vi "Tools Panel.vi"() -> ()   [LabVIEW 2019, in "Panther Dashboard.lvlib"]
uses:
  Panther Dashboard.lvlib
  <vilib>/PantherLAB/Panther Dashboard/Controls/Antidoc.ctl
  DQMH Tools Menu--enum.ctl
panel:
  in  "Add Event":bool caption="Add"
  in  "Remove Event":bool caption="Remove"
  in  "Convert Event":bool caption="Convert"
  in  "Rename Event":bool caption="Rename"
  in  "Open Documentation":bool caption="Open"
  in  "Generate Antidoc":T1 caption="Antidoc"
  in  "Add Module":bool caption="Add"
  in  "Rename Module":bool caption="Rename"
  in  "Validate Module":bool caption="Validate"
  in  "Create Module Template":bool caption="Template"
  in  "Add Unit Test":bool caption="Unit Test"
  in  "Create RT Tester":bool caption="RT Tester"
  in  "About":bool
  in  "Theme":bool
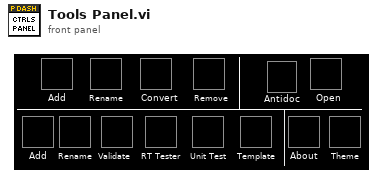
[diagram p1: front panel]
types:
  T1 = typedef "Antidoc.ctl" = bool
  T2 = typedef "Panther Dashboard.lvlib/Broadcast Events--cluster.ctl" = cluster{"Module Did Init":refnum<user-event>, "Status Updated":refnum<user-event>, "Error Reported":refnum<user-event>, "Module Did Stop":refnum<user-event>, "Update Module Execution Status":refnum<user-event>, "References Updated":refnum<user-event>, "Projects Updated":refnum<user-event>, "Targets Updated":refnum<user-event>, "Progress updated":refnum<user-event>, "Scale Updated":refnum<user-event>, "Connector Pane Updated":refnum<user-event>, "Documentation Updated":refnum<user-event>, "Module Type Updated":refnum<user-event>, "Theme Updated":refnum<user-event>, "Panel Position Updated":refnum<user-event>}
  T3 = typedef "Panther Dashboard.lvlib/DQMH Tools Menu--enum.ctl" = enum16{"Create New DQMH Event", "Remove DQMH Event", "Convert DQMH Event", "Rename DQMH Event", "Add New DQMH Module", "Create RT Tester", "Rename DQMH Module", "Validate DQMH Module", "Create DQMH Module Template", "New DQMH  Unit Test"}
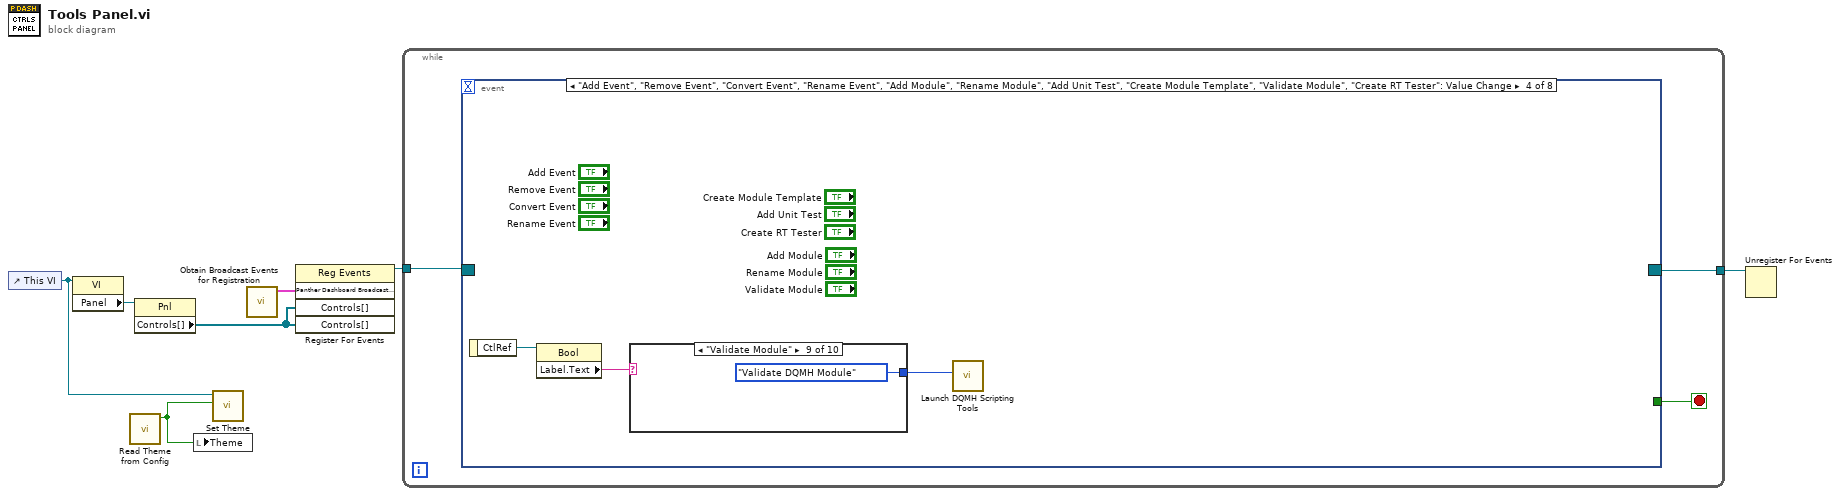
[diagram p0: block diagram]
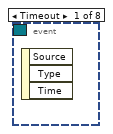
[diagram p2: hidden frame]
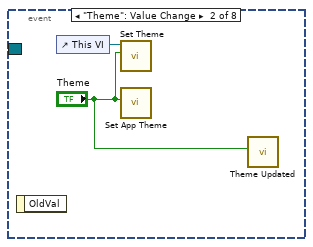
[diagram p3: hidden frame]
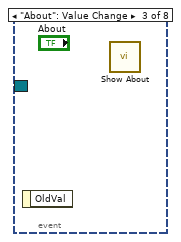
[diagram p4: hidden frame]
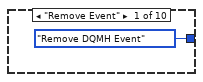
[diagram p5: hidden frame]
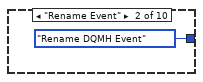
[diagram p6: hidden frame]
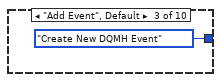
[diagram p7: hidden frame]
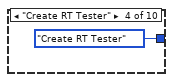
[diagram p8: hidden frame]
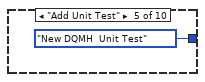
[diagram p9: hidden frame]
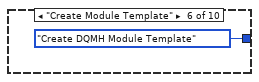
[diagram p10: hidden frame]
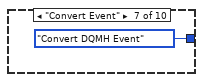
[diagram p11: hidden frame]
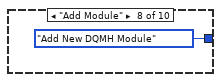
[diagram p12: hidden frame]
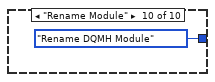
[diagram p13: hidden frame]
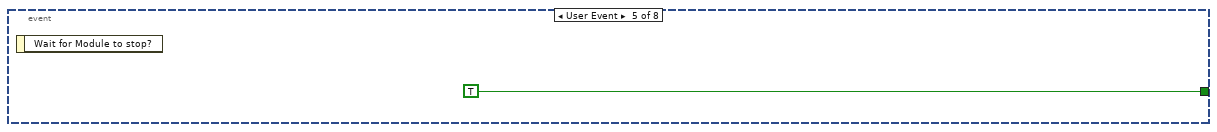
[diagram p14: hidden frame]
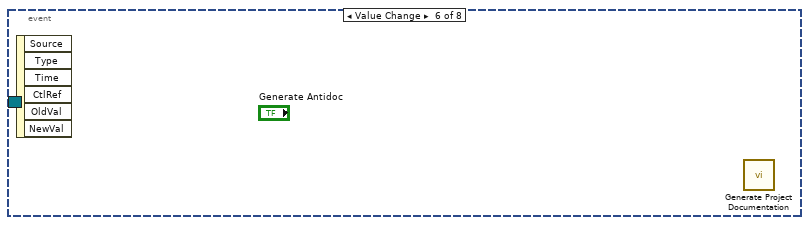
[diagram p15: hidden frame]
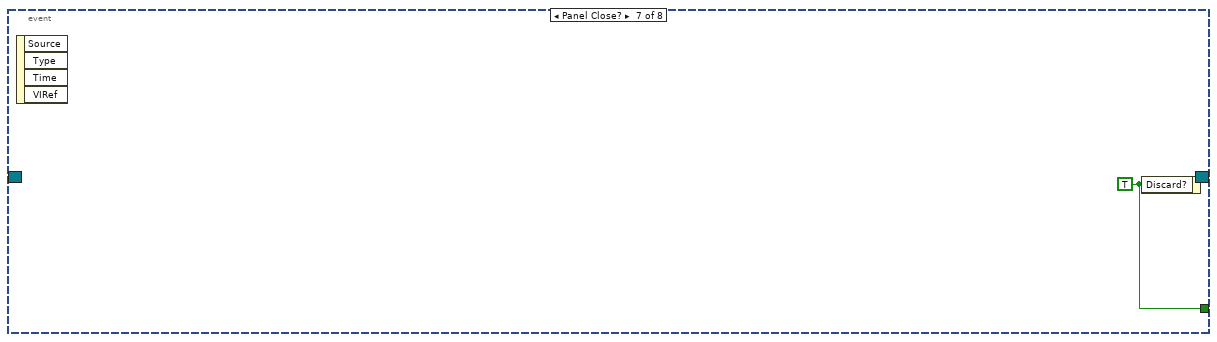
[diagram p16: hidden frame]
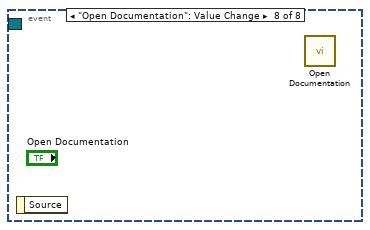
[diagram p17: hidden frame]
diagram:
  n1 = control-ref of="This VI"() -> (w4:refnum<vi>)
  n2 = property class="VI"(reference=w4) -> ("Panel"=w3:refnum<vi>)  [unwired: 1 in, 2 out]
  n3 = call "Read Theme from Config.vi"() -> ("Theme"=w1:bool)  [unwired: 10 in, 1 out]
  n4 = property class="Pnl"(reference=w3) -> ("Controls[]"=w2:refnum<vi>[])  [unwired: 1 in, 2 out]
  n5 = local write "Theme"(w1) -> ()
  n6 = call "Set Theme.vi"("Dark?"=w1, "VI in"=w4) -> ()  [unwired: 10 in]
  n7 = call "Obtain Broadcast Events for Registration.vi"() -> ("Panther Dashboard Broadcast Events"=w6:T2)  [unwired: 9 in, 2 out]
  n8 = register-events(w6, w2, w2) -> (reference out=w7:refnum<event-registration>)  [unwired: 2 in, 1 out]
  n9 = while {
    tunnel: w7 -> [w10]
    tunnel: [w8] -> w5
    stop <- w9 stop-if-true
    n10 = event shown="[3] \"Add Event\", \"Remove Event\", \"Convert Event\", \"Rename Event\", \"Add Module\", \"Rename Module\", \"Add Unit Test\", \"Create Module Template\", \"Validate Module\", \"Create RT Tester\": Value Change" {
      selector: w10 -> [_ _ _ _ _ _ _ _]
      dyn-events: [_ _ _ _ _ _ _ _] -> w8
      timeout: _ -> [_ _ _ _ _ _ _ _]
      tunnel: [_ _ _ _ TRUE _ w27 _] -> w9
      event Timeout {
        n11 = event-data() -> ()  [unwired: 1 in, 3 out]
      }
      event "Theme": Value Change {
        n12 = event-data() -> ()  [unwired: 1 in, 1 out]
        n13 = control-ref of="This VI"() -> (w12:refnum<vi>)
        n14 = call "Set Theme.vi"("Dark?"="Theme", "VI in"=w12) -> ()  [unwired: 10 in]
        n15 = call "Set App Theme.vi"("Theme"="Theme") -> ()  [unwired: 10 in, 1 out]
        n16 = call "Theme Updated.vi"("Theme"="Theme") -> ()  [unwired: 10 in, 1 out]
      }
      event "About": Value Change {
        n17 = event-data() -> ()  [unwired: 1 in, 1 out]
        n18 = call "Show About.vi"() -> ()  [unwired: 11 in, 1 out]
      }
      event "Add Event", "Remove Event", "Convert Event", "Rename Event", "Add Module", "Rename Module", "Add Unit Test", "Create Module Template", "Validate Module", "Create RT Tester": Value Change {
        n19 = event-data() -> ("CtlRef"=w15:refnum<vi>)  [unwired: 1 in]
        n20 = property class="Bool"(reference=w15) -> ("Label.Text"=w14:string)  [unwired: 1 in, 2 out]
        n21 = case shown="\"Validate Module\"" w14 {
          tunnel: [DQMH_Tools_Menu--enum."Remove DQMH Event" ("DQMH Tools") DQMH_Tools_Menu--enum."Rename DQMH Event" ("DQMH Tools") DQMH_Tools_Menu--enum."Create New DQMH Event" ("DQMH Tools") DQMH_Tools_Menu--enum."Create RT Tester" ("DQMH Tools") DQMH_Tools_Menu--enum."New DQMH  Unit Test" ("DQMH Tools") DQMH_Tools_Menu--enum."Create DQMH Module Template" ("DQMH Tools") DQMH_Tools_Menu--enum."Convert DQMH Event" ("DQMH Tools") DQMH_Tools_Menu--enum."Add New DQMH Module" ("DQMH Tools") DQMH_Tools_Menu--enum."Validate DQMH Module" ("DQMH Tools") DQMH_Tools_Menu--enum."Rename DQMH Module" ("DQMH Tools")] -> w13
          frame "Remove Event" {
          }
          frame "Rename Event" {
          }
          frame "Add Event", Default {
          }
          frame "Create RT Tester" {
          }
          frame "Add Unit Test" {
          }
          frame "Create Module Template" {
          }
          frame "Convert Event" {
          }
          frame "Add Module" {
          }
          frame "Validate Module" {
          }
          frame "Rename Module" {
          }
        }
        n22 = call "Launch DQMH Scripting Tools.vi"("Scripting Tool"=w13) -> ()  [unwired: 10 in, 1 out]
      }
      event User Event {
        n23 = event-data() -> ()  [unwired: 1 in, 1 out]
      }
      event Value Change {
        n24 = event-data() -> ()  [unwired: 1 in, 6 out]
        n25 = call "Generate Project Documentation.vi"() -> ()  [unwired: 11 in, 1 out]
      }
      event Panel Close? {
        w27 = TRUE ("Discard?")
        n26 = event-data() -> ()  [unwired: 1 in, 4 out]
        n27 = event-data("Discard?"=w27) -> ()  [unwired: 1 in, 1 out]
      }
      event "Open Documentation": Value Change {
        n28 = event-data() -> ()  [unwired: 1 in, 1 out]
        n29 = call "Open Documentation.vi"() -> ()  [unwired: 11 in, 1 out]
      }
    }
  }
  n30 = Unregister For Events(event registration refnum=w5) -> ()  [unwired: 1 in, 1 out]
